vi "UpdateIO.vi"(10 "IO Data":string[][](array[string]), 11 "MulticolumnListbox输入":refnum<vi>) -> (3 "大小":i32)   [LabVIEW 2017]
panel:
  out "转置的数组":string[][](array[string])
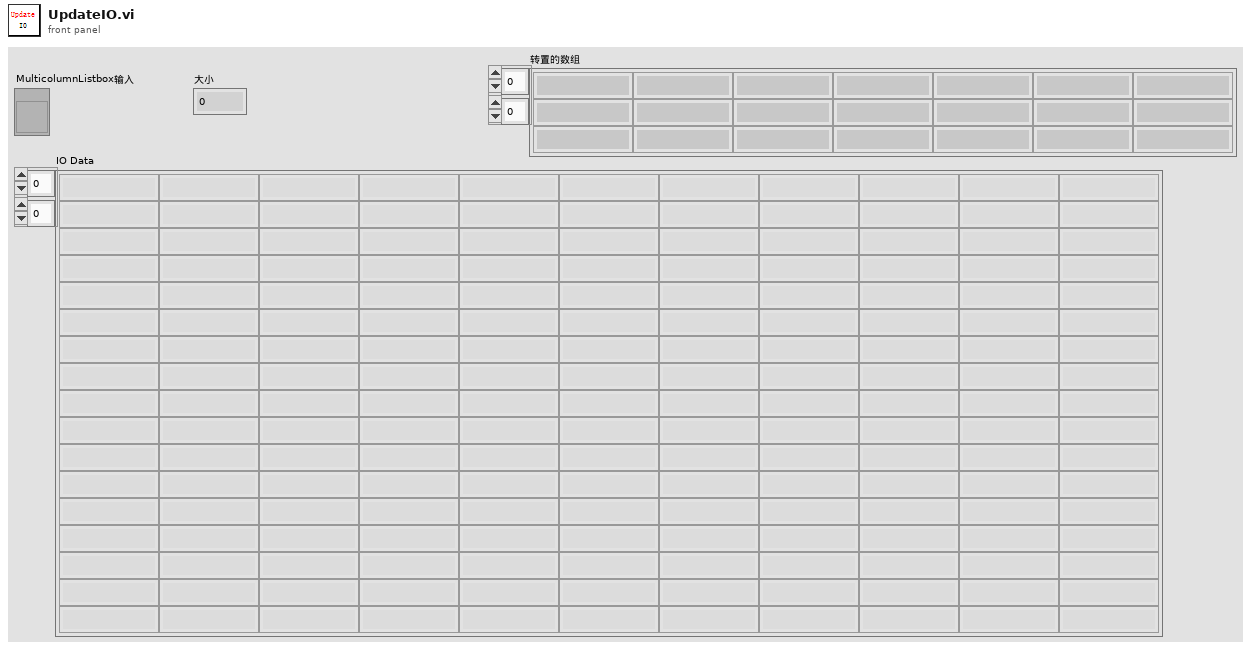
[diagram p1: front panel]
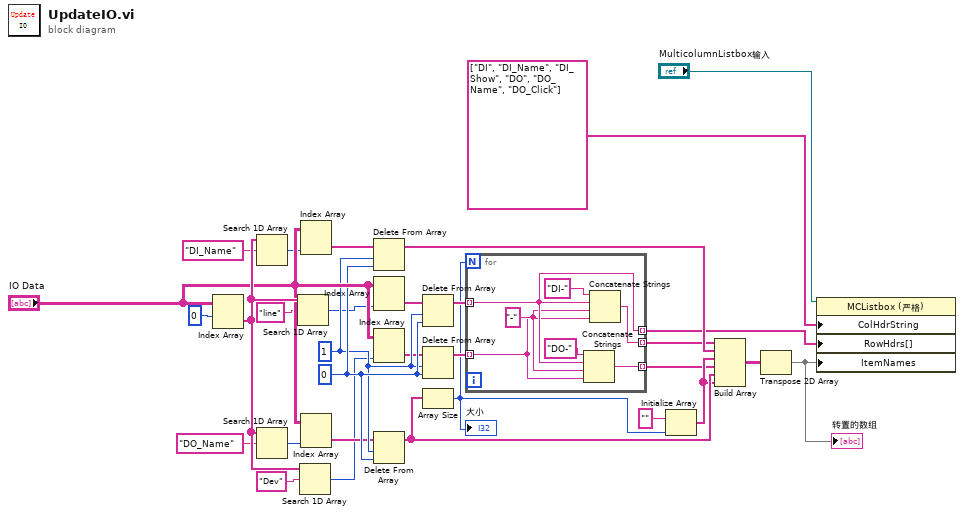
[diagram p0: block diagram]
diagram:
  w21 = 1 ("长度")
  w22 = 0 ("索引")
  n1 = Index Array(array="IO Data", index (row)=0 ("索引 (行)")) -> (element=w30:string[])  [unwired: 1 in]
  n2 = Search 1D Array(1D array=w30, element="DI_Name" ("元素")) -> (index of element=w20:i32)  [unwired: 1 in]
  n3 = Search 1D Array(1D array=w30, element="DO_Name" ("元素")) -> (index of element=w19:i32)  [unwired: 1 in]
  n4 = Search 1D Array(1D array=w30, element="line" ("元素")) -> (index of element=w7:i32)  [unwired: 1 in]
  n5 = Search 1D Array(1D array=w30, element="Dev" ("元素")) -> (index of element=w5:i32)  [unwired: 1 in]
  n6 = Index Array(array="IO Data", index (col)=w20) -> (element=w18:string[])  [unwired: 1 in]
  n7 = Index Array(array="IO Data", index (col)=w19) -> (element=w17:string[])  [unwired: 1 in]
  n8 = Delete From Array(array=w18, length=w21, index=w22) -> (array with subset deleted=w16:string[])  [unwired: 1 out]
  n9 = Index Array(array="IO Data", index (col)=w7) -> (element=w8:string[])  [unwired: 1 in]
  n10 = Index Array(array="IO Data", index (col)=w5) -> (element=w4:string[])  [unwired: 1 in]
  n11 = Delete From Array(array=w17, length=w21, index=w22) -> (array with subset deleted=w15:string[])  [unwired: 1 out]
  n12 = Delete From Array(array=w8, length=w21, index=w22) -> (array with subset deleted=w6:string[])  [unwired: 1 out]
  n13 = Delete From Array(array=w4, length=w21, index=w22) -> (array with subset deleted=w3:string[])  [unwired: 1 out]
  n14 = Array Size(array=w15) -> (size(s)=w2:i32)
  "大小" <- w2
  n15 = for {
    N: w2 -> [_]
    tunnel: [w34] -> w11 mode=indexing
    tunnel: [w37] -> w9 mode=indexing
    tunnel: [w35] -> w10 mode=indexing
    tunnel: w6 -> [w34] mode=indexing
    tunnel: w3 -> [w32] mode=indexing
    w33 = "-" ("字符串")
    n16 = Concatenate Strings("DO-", w34, w33, w32) -> (w35:string)
    n17 = Concatenate Strings("DI-", w34, w33, w32) -> (w37:string)
  }
  n18 = Initialize Array("", w2) -> (w14:string[])
  n19 = Build Array(w9, w16, w14, w10, w15, w14) -> (w13:string[][])
  n20 = Transpose 2D Array(2D array=w13) -> (transposed array=w12:string[][])
  "转置的数组" <- w12
  n21 = property class="MCListbox (严格)"(reference="MulticolumnListbox输入", "ColHdrString"=string[] ["DI", "DI_Name", "DI_Show", "DO", "DO_Name", "DO_Click"] ("列首字符串[]"), "RowHdrs[]"=w11, "ItemNames"=w12) -> ()  [unwired: 1 in, 2 out]
